vi "Get User Interface Details.vi"(8 "error in":errorcluster, 11 "measurement plugin service in":refnum<class "Measurement Plugin Service.lvclass">) -> (0 "error out":errorcluster, 2 "user interface details":T1[](array[typedef]), 3 "measurement plugin service out":refnum<class "Measurement Plugin Service.lvclass">)   [LabVIEW 2021, in "NI Measurement Plug-In SDK.lvlib" / "Measurement Plugin Service.lvclass"]
doc: "Provides information about the user interfaces supported by the measurement if any. The user interface file is specified as a file URL."
uses:
  Measurement Plugin Service.lvclass
  Helpers/TypeDefs/User Interface Details.ctl
  Helpers/TypeDefs/User Interface Information.ctl
  <vilib>/regexp/Match Regular Expression.xnode
  NI Measurement Plug-In SDK.lvlib
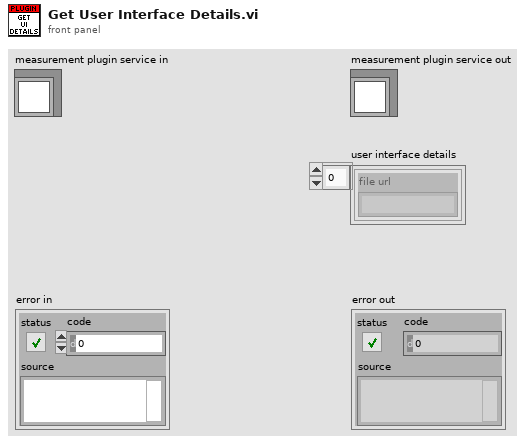
[diagram p1: front panel]
types:
  T1 = typedef "NI Measurement Plug-In SDK.lvlib/User Interface Details.ctl" = cluster{"file url":string}
  T2 = typedef "NI Measurement Plug-In SDK.lvlib/Measurement Plugin Service.lvclass/Plugin Paths.ctl" = cluster{"get service descriptor VI path":path, "get type specializations VI path":path, "get UI details VI path":path, "measurement logic VI path":path, "measurement configuration ctl path":path, "measurement results ctl path":path}
  T3 = typedef "NI Measurement Plug-In SDK.lvlib/User Interface Information.ctl" = cluster{"file":string}
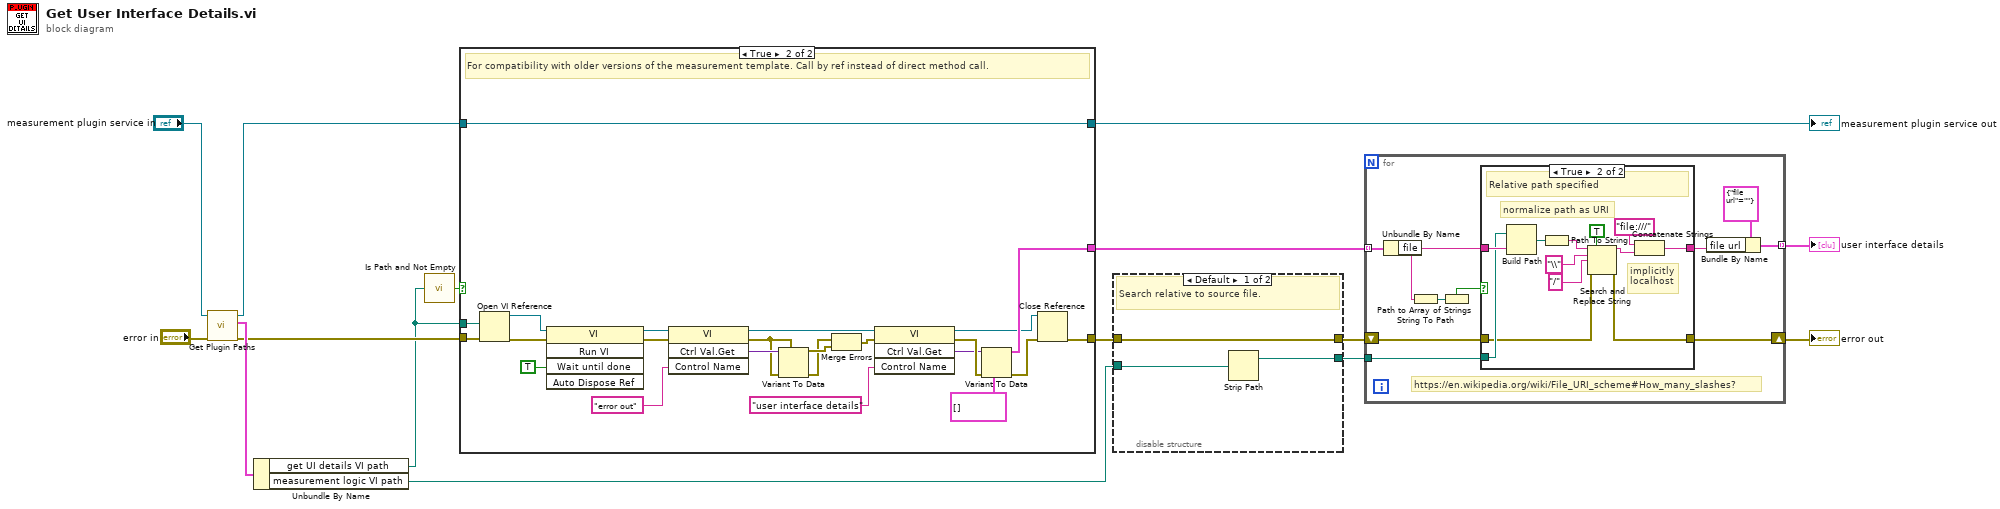
[diagram p0: block diagram]
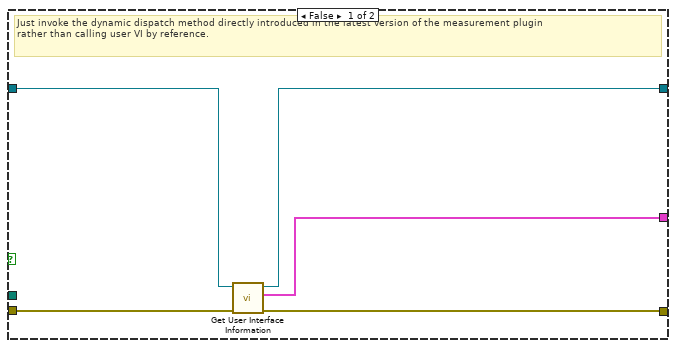
[diagram p2: hidden frame]
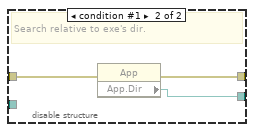
[diagram p3: hidden frame]
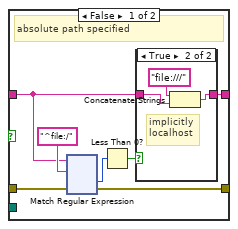
[diagram p4: hidden frame]
diagram:
  n1 = call-dynamic "Get Plugin Paths.vi"("error in"="error in", "measurement plugin service in"="measurement plugin service in") -> ("error out"=w11:errorcluster, "plugin paths"=w12:T2, "measurement plugin service out"=w3:refnum<class "Measurement Plugin Service.lvclass">)  [unwired: 7 in]
  n2 = Unbundle By Name(w12) -> ("get UI details VI path"=w5:path, "measurement logic VI path"=w6:path)
  n3 = call <vilib>:"Is Path and Not Empty.vi"("path"=w5) -> ("Is Path and Not Empty?"=w4:bool)  [unwired: 4 in]
  n4 = case shown="True" w4 {
    tunnel: w11 -> [w19 w43]
    tunnel: [w16 w30] -> w2
    tunnel: [w17 w24] -> w7
    tunnel: w5 -> [_ w22]
    tunnel: w3 -> [w20 w21]
    tunnel: [w18 w21] -> w1
    frame False {
      # "Just invoke the dynamic dispatch method directly introduced in the latest version of the measurement plugin\nrather than calling user VI by reference."
      n5 = call-dynamic "Get User Interface Information.vi"("error in (no error)"=w19, "measurement plugin service in"=w20) -> ("error out"=w17:errorcluster, "user interface information"=w16:T3[], "measurement plugin service out"=w18:refnum<class "Measurement Plugin Service.lvclass">)  [unwired: 7 in]
    }
    frame True {
      # "For compatibility with older versions of the measurement template. Call by ref instead of direct method call."
      n6 = Open VI Reference(vi path=w22, error in (no error)=w43) -> (vi reference=w26:refnum<vi>, error out=w27:errorcluster)  [unwired: 4 in]
      n7 = invoke class="VI" method="Run VI"(reference=w26, error in=w27, "Wait until done"=TRUE ("Wait Until Done")) -> (reference out=w33:refnum<vi>, error out=w32:errorcluster)  [unwired: 2 in, 3 out]
      n8 = invoke class="VI" method="Ctrl Val.Get"(reference=w33, error in=w32, "Control Name"="error out") -> (reference out=w29:refnum<vi>, error out=w38:errorcluster, "Get Control Value Variant"=w39:variant)  [unwired: 1 in, 1 out]
      n9 = Variant To Data(error in=w38, type=w38, Variant=w39) -> (data=w37:errorcluster, error out=w28:errorcluster)
      n10 = Merge Errors(w28, w37) -> (w31:errorcluster)
      n11 = invoke class="VI" method="Ctrl Val.Get"(reference=w29, error in=w31, "Control Name"="user interface details") -> (reference out=w23:refnum<vi>, error out=w36:errorcluster, "Get Control Value Variant"=w34:variant)  [unwired: 1 in, 1 out]
      n12 = Variant To Data(error in=w36, type=T3[] [], Variant=w34) -> (data=w30:T3[], error out=w25:errorcluster)
      n13 = Close Reference(reference=w23, error in (no error)=w25) -> (error out=w24:errorcluster)
    }
  }
  "measurement plugin service out" <- w1
  n14 = disable-structure shown="Default" {
    disable-tunnel: w7 -> [w44 w49]
    disable-tunnel: [w44 w48] -> w8
    disable-tunnel: [w46 w47] -> w9
    disable-tunnel: w6 -> [w45 _]
    frame condition #0 (active) {
      # "Search relative to source file."
      n15 = Strip Path(path=w45) -> (stripped path=w46:path)  [unwired: 1 out]
    }
    frame condition #1 {
      # "Search relative to exe's dir."
      n16 = property class="App"(error in=w49) -> (error out=w48:errorcluster, "App.Dir"=w47:path)  [unwired: 1 in, 1 out]
    }
  }
  n17 = for {
    tunnel: w2 -> [w57] mode=indexing
    tunnel: [w58] -> w13 mode=indexing
    shift-right: [w50] -> w10
    shift-left: w8 -> [w51]
    tunnel: w9 -> [w54]
    # "https://en.wikipedia.org/wiki/File_URI_scheme#How_many_slashes?"
    n18 = Unbundle By Name(w57) -> ("file"=w53:string)
    n19 = String To Path(string=w53) -> (path=w56:path)
    n20 = Path to Array of Strings(0:w56) -> (1:w55:bool)  [unwired: 1 out]
    n21 = case shown="True" w55 {
      tunnel: w54 -> [_ w198]
      tunnel: w53 -> [w62 w199]
      tunnel: [w61 w195] -> w52
      tunnel: w51 -> [w65 w189]
      tunnel: [w60 w188] -> w50
      frame False {
        # "absolute path specified"
        n22 = xnode "Match Regular Expression"("input string"=w62, "regular expression"="^file:/", "error in"=w65) -> ("offset past match"=w64:i32, "error out"=w60:errorcluster)  [unwired: 3 in, 3 out]
        n23 = Less Than 0?(x=w64) -> (x < 0?=w63:bool)
        n24 = case shown="True" w63 {
          tunnel: w62 -> [w67 w69]
          tunnel: [w67 w68] -> w61
          frame False {
            # "already uri.\npreserve it"
          }
          frame True {
            # "implicitly\nlocalhost"
            n25 = Concatenate Strings("file:///" ("string"), w69) -> (w68:string)
          }
        }
      }
      frame True {
        # "normalize path as URI"
        # "implicitly\nlocalhost"
        # "Relative path specified"
        n26 = Build Path(base path=w198, name or relative path=w199) -> (appended path=w197:path)
        n27 = Path To String(path=w197) -> (string=w193:string)
        n28 = Search and Replace String(replace all?=TRUE ("replace all? (F)"), input string=w193, search string="\\", replace string="/" ("replace string (\"\")"), error in=w189) -> (result string=w190:string, error out=w188:errorcluster)  [unwired: 3 in, 2 out]
        n29 = Concatenate Strings("file:///" ("string"), w190) -> (w195:string)
      }
    }
    n30 = Bundle By Name(cluster=T1 {"file url"=""} ("UserInterfaceDetails"), "file url"=w52) -> (w58:T1)
  }
  "error out" <- w10
  "user interface details" <- w13
